vi "Data_DisplayChange.vi"(1 "显示方式":u16(ring) items=["原始显示", "拆分显示"], 9 "data0":dbl[][](array[numeric])) -> (10 "2D data":dbl[][](array[numeric]))   [LabVIEW 2013]
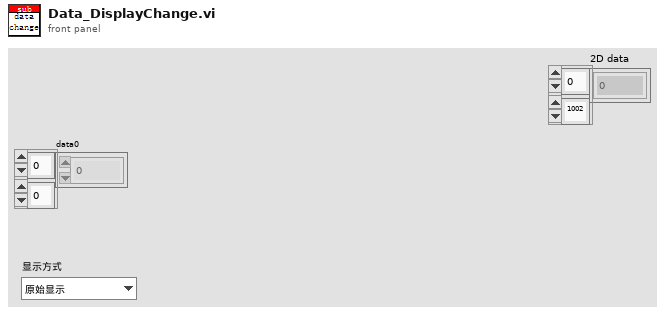
[diagram p1: front panel]
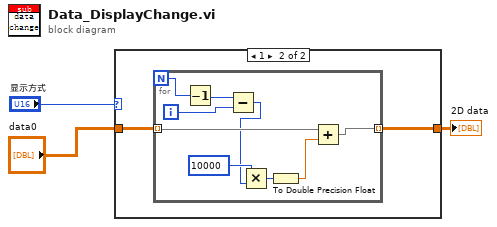
[diagram p0: block diagram]
diagram:
  n1 = case shown="1" "显示方式" {
    tunnel: "data0" -> [w4 w6]
    tunnel: [w4 w5] -> w2
    frame 0, Default {
    }
    frame 1 {
      n2 = for {
        N -> [w10]
        tunnel: w6 -> [w15] mode=indexing
        tunnel: [w11] -> w5 mode=indexing
        i -> [w8]
        n3 = Decrement(x=w10) -> (x-1=w9:i32)
        n4 = Subtract(x=w9, y=w8) -> (x-y=w7:i32)
        n5 = Multiply(x=10000, y=w7) -> (x*y=w13:i32)
        n6 = To Double Precision Float(number=w13) -> (double precision float=w12:dbl)
        n7 = Add(x=w15, y=w12) -> (x+y=w11:dbl[])
      }
    }
  }
  "2D data" <- w2
